vi "Global Data!!!.vi"() -> ()   [LabVIEW 2014]
panel:
  in  "OutTotesRC":bool
  in  "Intake":dbl
  in  "just to be sure":bool
  in  "ResetFeederMode":bool
  in  "FeederMode?":bool
  in  "resetDesired":bool
  in  "TransitionComplete?":bool
  in  "RCReset":bool
  in  "RC?":bool
  in  "ArmsOut?":bool
  in  "LiftSpeed":dbl
  in  "FromAuto":bool
  in  "Stage2?":bool
  in  "Stage1?":bool
  in  "inManual?":bool
  out "mainState":i8
  in  "resetDriveEnc":bool
  in  "gyroAngleForAuto":dbl
  in  "manualRESET!!!!!!!!!!!!!!":bool
  in  "outTotesButton":bool
  in  "desiredEncoderValue":dbl
  in  "targetLocation":dbl
  in  "manualElevatorReLevel?":bool
  in  "manualElevatorDown":bool
  in  "manualElevatorUp":bool
  in  "buttonCount":bool
  in  "dropButton":bool
  in  "elevatorActive":bool
  in  "autoLift":bool
  in  "2StageButton":bool
  in  "intakeSensor":bool
  in  "Reset":bool
  in  "bottomBrake":bool
  in  "testRIght":dbl
  in  "testLeft":dbl
  in  "Testing":dbl
  in  "1StagePneumaticsButton":bool
  in  "liftEnc":dbl
  in  "sixInch":bool
  in  "desiredLevel":dbl=1.0
  in  "interruptUp":bool
  in  "stack":bool
  in  "outTotes":bool
  in  "lift1Stage":bool
  in  "manual?":bool
  in  "rightEnc":dbl
  in  "leftEnc":dbl
  in  "resetLift?":bool
  in  "secondStagePneumatics":bool
  in  "firstStagePneumatics":bool
  in  "elevatorLift":dbl
  in  "gyroAngle":dbl
  in  "straightDrive":bool
  in  "Turn":dbl
  in  "Power":dbl
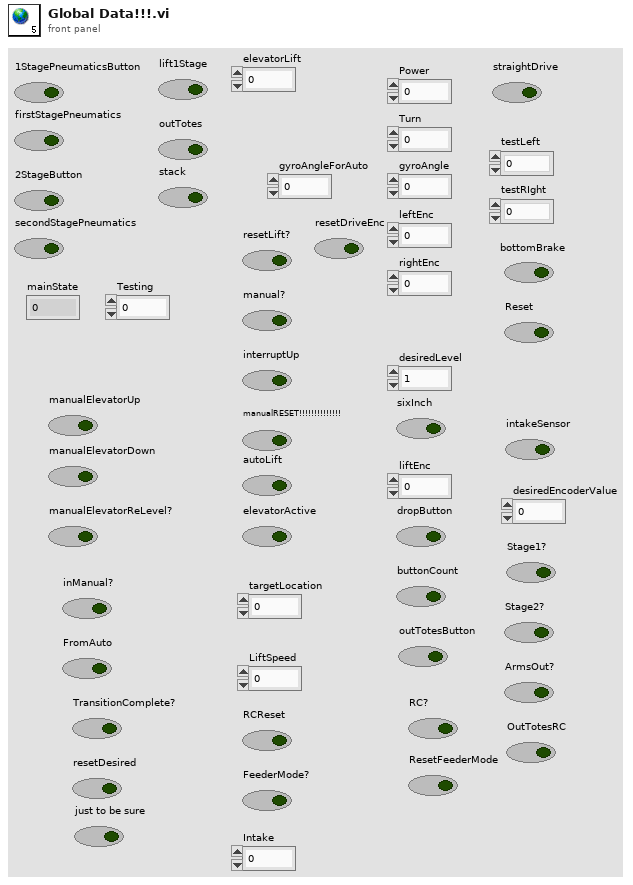
[diagram p1: front panel]
diagram:
